vi "Maquina_Sondeo.vi"() -> ()   [LabVIEW 2016]
uses:
  Control1_Enum.ctl
panel:
  in  "Paro":bool
  out "MD":bool
  out "MI":bool
  in  "S":bool
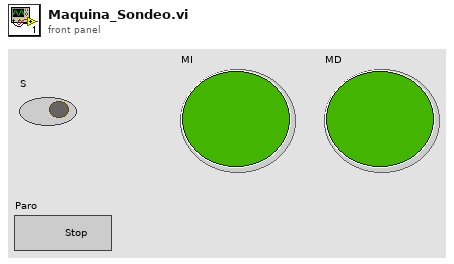
[diagram p1: front panel]
types:
  T1 = typedef "Control1_Enum.ctl" = enum16{"Avance 1", "Avance2", "Giro Izquierda", "Giro Derecha", "Paro"}
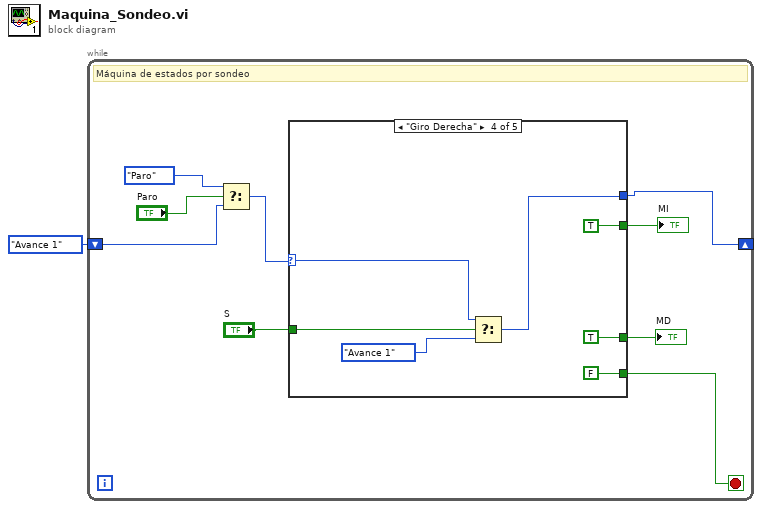
[diagram p0: block diagram]
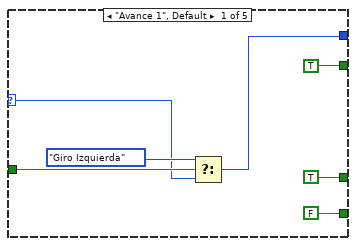
[diagram p2: hidden frame]
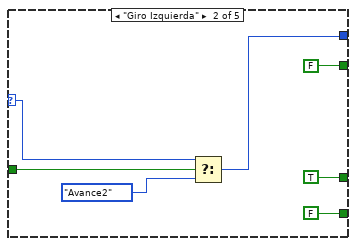
[diagram p3: hidden frame]
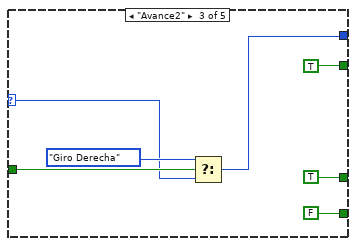
[diagram p4: hidden frame]
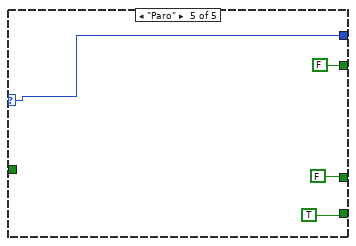
[diagram p5: hidden frame]
diagram:
  n1 = while {
    shift-right: [w7] -> _
    shift-left: Control1_Enum."Avance 1" -> [w4]
    stop <- w6 stop-if-true
    # "Máquina de estados por sondeo"
    n2 = Select(t=Control1_Enum."Paro", s="Paro", f=w4) -> (s? t:f=w2:T1)
    n3 = case shown="\"Giro Derecha\"" w2 {
      selector: w2 -> [w11 w18 w25 w32 w40]
      tunnel: "S" -> [w17 w24 w31 w38 _]
      tunnel: [w16 w23 w30 w37 w40] -> w7
      tunnel: [FALSE FALSE FALSE FALSE TRUE] -> w6
      tunnel: [TRUE TRUE TRUE TRUE FALSE] -> w9
      tunnel: [TRUE FALSE TRUE TRUE FALSE] -> w10
      frame "Avance 1", Default {
        n4 = Select(t=Control1_Enum."Giro Izquierda", s=w17, f=w11) -> (s? t:f=w16:T1)
      }
      frame "Giro Izquierda" {
        n5 = Select(t=w18, s=w24, f=Control1_Enum."Avance2") -> (s? t:f=w23:T1)
      }
      frame "Avance2" {
        n6 = Select(t=Control1_Enum."Giro Derecha", s=w31, f=w25) -> (s? t:f=w30:T1)
      }
      frame "Giro Derecha" {
        n7 = Select(t=w32, s=w38, f=Control1_Enum."Avance 1") -> (s? t:f=w37:T1)
      }
      frame "Paro" {
      }
    }
    "MI" <- w10
    "MD" <- w9
  }
